vi "Failed Test Counter.vi"(8 "error in (no error)":errorcluster, 9 "Result":bool, 10 "String":string, 11 "Boolean in":refnum<vi>) -> (0 "error out":errorcluster)   [LabVIEW 2013]
uses:
  Controls/FailedTests.ctl
  <vilib>/Utility/config.llb/NI_LVConfig.lvlib
  <vilib>/Utility/config.llb/Write Key (I32).vi
  <vilib>/Utility/config.llb/Read Key (I32).vi
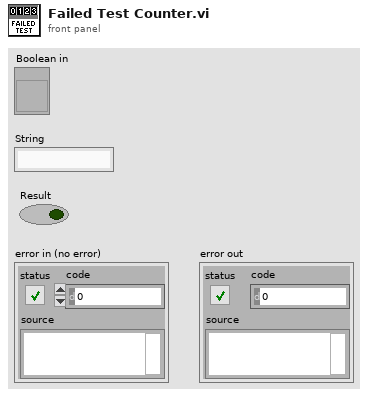
[diagram p1: front panel]
types:
  T1 = typedef "FailedTests.ctl" = enum16{"Initialize", "Add Serial", "Get Serial", "Remove Serial", "Close Config File"}
  T2 = typedef "NI_LVConfig.lvlib/Config Data RefNum.ctl" = refnum<k1>
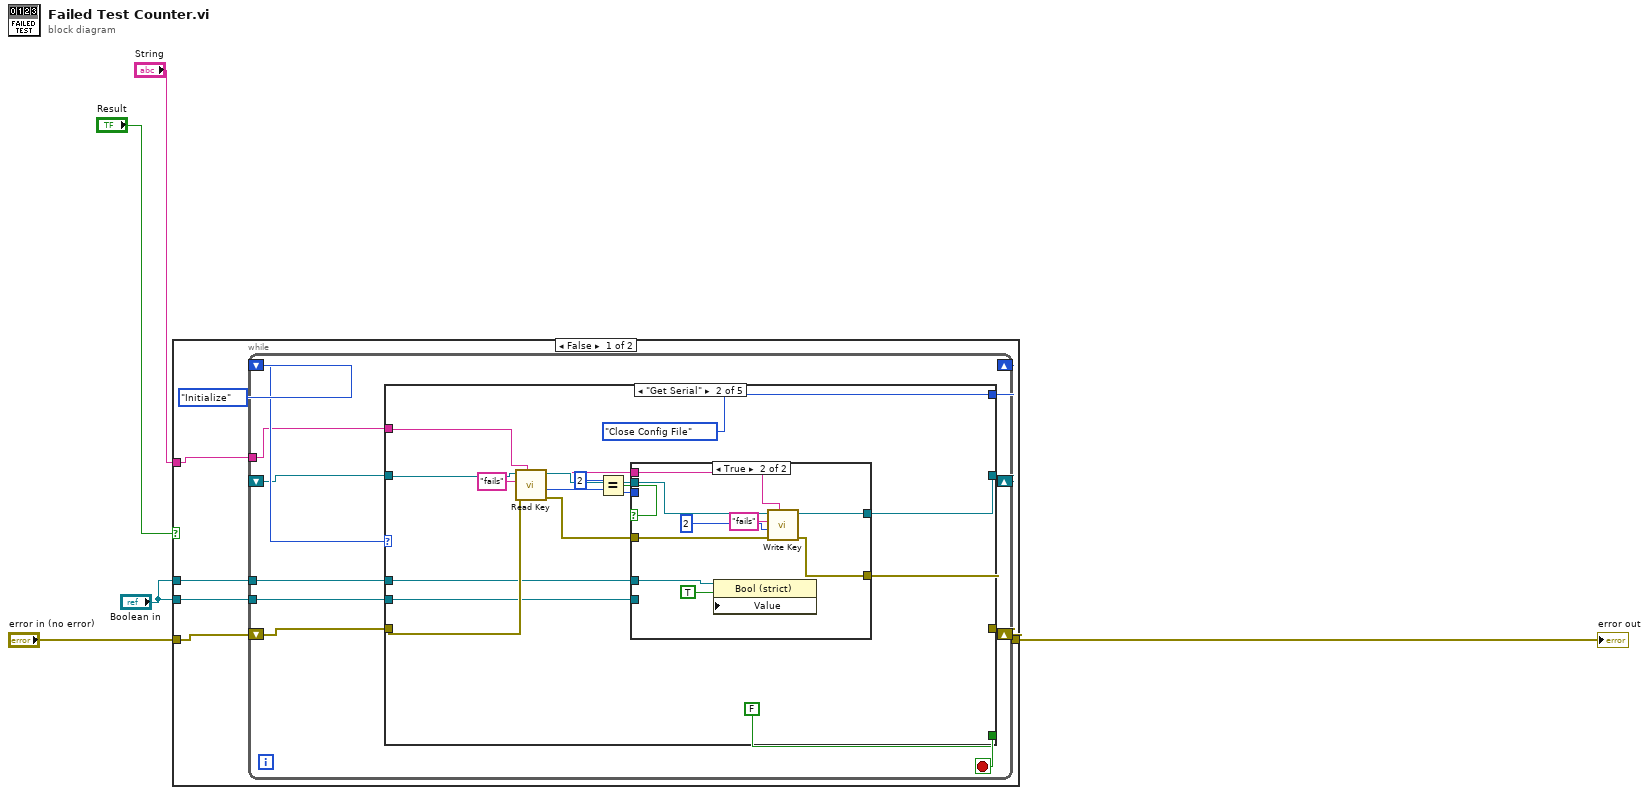
[diagram p0: block diagram]
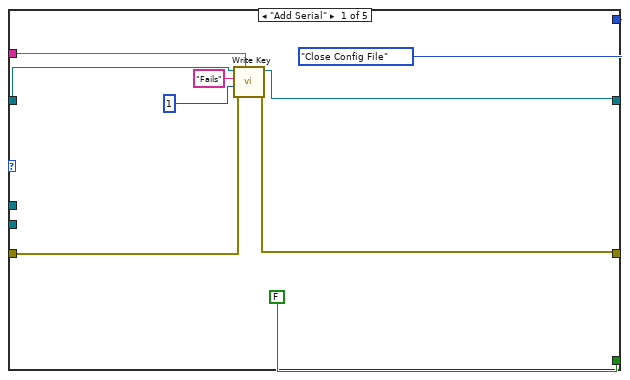
[diagram p2: hidden frame]
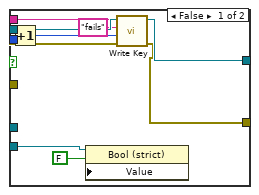
[diagram p3: hidden frame]
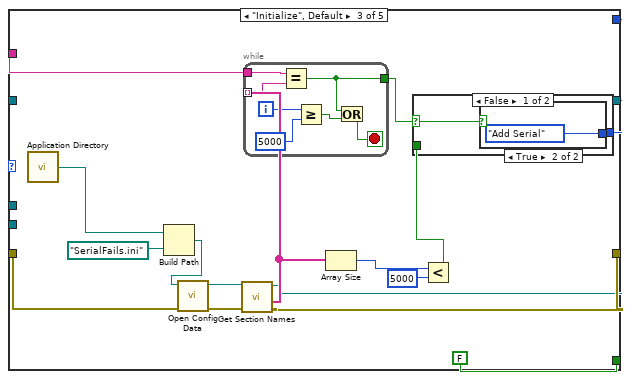
[diagram p4: hidden frame]
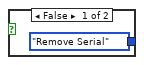
[diagram p5: hidden frame]
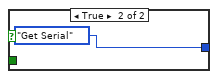
[diagram p6: hidden frame]
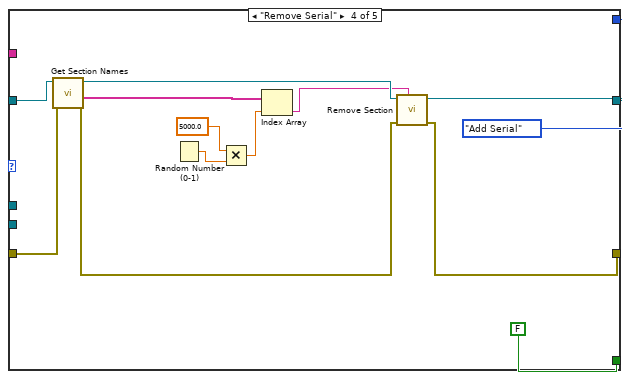
[diagram p7: hidden frame]
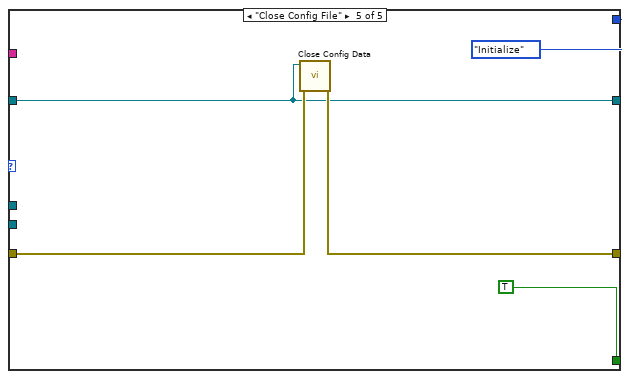
[diagram p8: hidden frame]
diagram:
  n1 = case shown="False" "Result" {
    tunnel: "error in (no error)" -> [w10 w111]
    tunnel: "String" -> [w9 _]
    tunnel: [w8 w111] -> w5
    tunnel: "Boolean in" -> [w7 _]
    tunnel: "Boolean in" -> [w6 _]
    frame False {
      n2 = while {
        shift-right: [w16] -> _
        shift-left: FailedTests."Initialize" -> [w21]
        shift-right: [w18] -> w8
        shift-left: w10 -> [w20]
        shift-right: [w19] -> _
        shift-left: _ -> [w15]
        tunnel: w9 -> [w17]
        tunnel: w7 -> [w13]
        tunnel: w6 -> [w12]
        stop <- w14 stop-if-true
        n3 = case shown="\"Remove Serial\"" w21 {
          tunnel: w20 -> [w29 w44 w80 w104 w110]
          tunnel: [w25 w37 w69 w94 w106] -> w19
          tunnel: [w24 w36 w77 w95 w109] -> w18
          tunnel: w17 -> [w28 w38 w76 _ _]
          tunnel: [FailedTests."Close Config File" FailedTests."Close Config File" w71 FailedTests."Add Serial" FailedTests."Initialize"] -> w16
          tunnel: w15 -> [w30 w45 _ w105 w106]
          tunnel: [FALSE FALSE FALSE FALSE TRUE] -> w14
          tunnel: w13 -> [_ w32 _ _ _]
          tunnel: w12 -> [_ w31 _ _ _]
          frame "Add Serial" {
            n4 = call-poly <vilib>:"Write Key.vi"("section"=w28, "error in (no error)"=w29, "value"=1, "key"="Fails", "refnum"=w30) -> ("error out"=w24:errorcluster, "refnum out"=w25:T2)  [unwired: 4 in, 1 out]
          }
          frame "Get Serial" {
            n5 = call-poly <vilib>:"Read Key.vi"("section"=w38, "error in (no error)"=w44, "key"="fails", "refnum"=w45) -> ("error out"=w39:errorcluster, "value"=w35:i32, "refnum out"=w40:T2)  [unwired: 4 in, 1 out]
            n6 = Equal?(x=2, y=w35) -> (x = y?=w41:bool)
            n7 = case shown="True" w41 {
              tunnel: w40 -> [w55 w63]
              tunnel: w39 -> [w54 w62]
              tunnel: w38 -> [w50 w60]
              tunnel: [w49 w59] -> w37
              tunnel: [w48 w58] -> w36
              tunnel: w35 -> [w53 _]
              tunnel: w32 -> [w46 _]
              tunnel: w31 -> [_ w56]
              frame False {
                n8 = Increment(x=w53) -> (x+1=w52:i32)
                n9 = property class="Bool (strict)"(reference=w46, "Value"=FALSE ("Unit failed 3x Tests")) -> ()  [unwired: 1 in, 2 out]
                n10 = call-poly <vilib>:"Write Key.vi"("section"=w50, "error in (no error)"=w54, "value"=w52, "key"="fails", "refnum"=w55) -> ("error out"=w48:errorcluster, "refnum out"=w49:T2)  [unwired: 4 in, 1 out]
              }
              frame True {
                n11 = property class="Bool (strict)"(reference=w56, "Value"=TRUE ("Unit failed 3x Tests")) -> ()  [unwired: 1 in, 2 out]
                n12 = call-poly <vilib>:"Write Key.vi"("section"=w60, "error in (no error)"=w62, "value"=2 ("x"), "key"="fails", "refnum"=w63) -> ("error out"=w58:errorcluster, "refnum out"=w59:T2)  [unwired: 4 in, 1 out]
              }
            }
          }
          frame "Initialize", Default {
            n13 = call <vilib>:"Application Directory.vi"() -> ("Application Directory"=w68:path)
            n14 = Build Path(base path=w68, name or relative path=path "SerialFails.ini") -> (appended path=w66:path)
            n15 = call <vilib>:"Open Config Data.vi"("error in (no error)"=w80, "configuration file path"=w66) -> ("error out"=w78:errorcluster, "refnum"=w79:T2)  [unwired: 7 in, 1 out]
            n16 = call <vilib>:"Get Section Names.vi"("error in (no error)"=w78, "refnum"=w79) -> ("error out"=w77:errorcluster, "section names"=w75:string[], "refnum out"=w69:T2)  [unwired: 7 in]
            n17 = while {
              tunnel: w75 -> [w92] mode=indexing
              tunnel: w76 -> [w91]
              tunnel: [w87] -> w72
              i -> [w90]
              stop <- w88 stop-if-true
              n18 = Equal?(x=w91, y=w92) -> (x = y?=w87:bool)
              n19 = Greater Or Equal?(x=w90, y=5000) -> (x >= y?=w86:bool)
              n20 = Or(x=w87, y=w86) -> (x .or. y?=w88:bool)
            }
            n21 = Array Size(array=w75) -> (size(s)=w74:i32)
            n22 = Less?(x=w74, y=5000) -> (x < y?=w70:bool)
            n23 = case shown="False" w72 {
              tunnel: [w81 FailedTests."Get Serial"] -> w71
              tunnel: w70 -> [w82 _]
              frame False {
                n24 = case shown="True" w82 {
                  tunnel: [FailedTests."Remove Serial" FailedTests."Add Serial"] -> w81
                  frame False {
                  }
                  frame True {
                  }
                }
              }
              frame True {
              }
            }
          }
          frame "Remove Serial" {
            n25 = call <vilib>:"Get Section Names.vi"("error in (no error)"=w104, "refnum"=w105) -> ("error out"=w97:errorcluster, "section names"=w102:string[], "refnum out"=w98:T2)  [unwired: 7 in]
            n26 = Random Number (0-1)() -> (number: 0 to 1=w101:dbl)
            n27 = Multiply(x=5000.0, y=w101) -> (x*y=w99:dbl)
            n28 = Index Array(array=w102, index=w99) -> (element=w96:string)
            n29 = call <vilib>:"Remove Section.vi"("section"=w96, "error in (no error)"=w97, "refnum"=w98) -> ("error out"=w95:errorcluster, "refnum out"=w94:T2)  [unwired: 6 in, 1 out]
          }
          frame "Close Config File" {
            n30 = call <vilib>:"Close Config Data.vi"("error in (no error)"=w110, "refnum"=w106) -> ("error out"=w109:errorcluster)  [unwired: 8 in, 1 out]
          }
        }
      }
    }
    frame True {
    }
  }
  "error out" <- w5
